vi "Write Process SV.vi"(8 "error in (no error)":errorcluster, 10 "Process SV":dbl format="%.2f", 11 "EMKO in":refnum<class "ESM-xx50.lvclass">) -> (0 "error out":errorcluster, 3 "EMKO out":refnum<class "ESM-xx50.lvclass">)   [LabVIEW 2023, in "EMKO.lvlib" / "ESM-xx50.lvclass"]
uses:
  ESM-xx50.lvclass
  ESM-xx50.lvclass/ESM-xx50.ctl
  <vilib>/Modbus/master/Modbus Master.lvclass
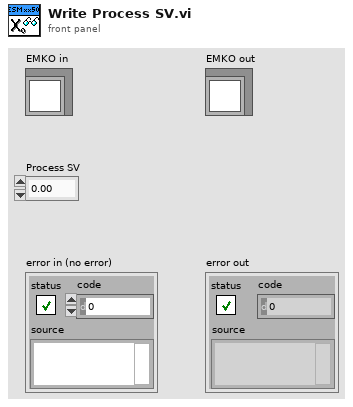
[diagram p1: front panel]
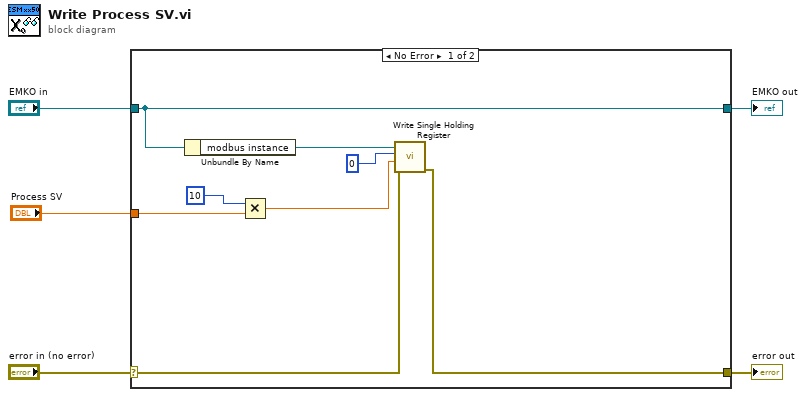
[diagram p0: block diagram]
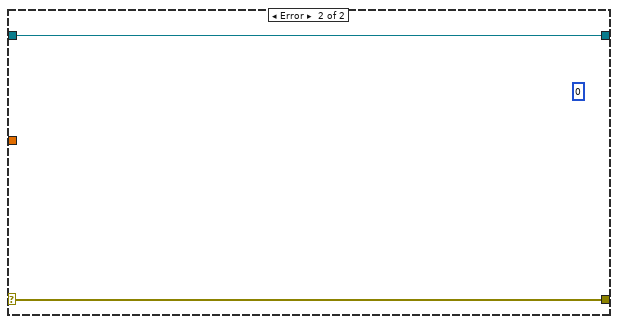
[diagram p2: hidden frame]
diagram:
  n1 = case shown="No Error" "error in (no error)" {
    selector: "error in (no error)" -> [w8 w15]
    tunnel: [w9 w15] -> w4
    tunnel: [w13 w14] -> w2
    tunnel: "EMKO in" -> [w13 w14]
    tunnel: "Process SV" -> [w11 _]
    frame No Error {
      n2 = Unbundle By Name(w13) -> ("modbus instance"=w6:refnum<class "Modbus Master.lvclass">)
      n3 = Multiply(x=u16 10 ("y"), y=w11) -> (x*y=w7:dbl)
      n4 = call-dynamic "Write Single Holding Register.vi"("error in (no error)"=w8, "holding register value"=w7, "address"=u16 0 ("starting address"), "Modbus master in"=w6) -> ("error out"=w9:errorcluster)  [unwired: 6 in, 1 out]
    }
    frame Error {
      (unwired) u16 0 ("register")
    }
  }
  "error out" <- w4
  "EMKO out" <- w2
